vi "Get Peaks.vi"(8 "error in (no error)":errorcluster, 11 "Micron Hyperion Driver in":refnum<class "Micron Hyperion Driver.lvclass">) -> (0 "error out":errorcluster, 1 "Peaks per channel":i32[](array[numeric]), 2 "Peaks":dbl[](array[numeric]), 3 "Micron Hyperion Driver out":refnum<class "Micron Hyperion Driver.lvclass">)   [LabVIEW 2016, in "Micron Hyperion Driver.lvclass"]
uses:
  Micron Hyperion Driver.lvclass
  C:/github/NHMFL_Core/Libraries/Instruments/Micron Optics/Micron Optics Driver/Micron Optics Driver.lvclass
  C:/github/NHMFL_Core/Libraries/Instruments/Instrument Driver/Instrument Driver.lvclass
  Instrument Driver/Instrument Driver.lvclass/Instrument Driver.ctl
  Micron Optics Driver/Micron Optics Driver.lvclass/Micron Optics Driver.ctl
  Micron Optics Driver/Read Peaks buffer.vi
  Micron Optics Driver/Read Number of peaks.vi
  Instrument Driver/Read Cycle period.vi
  Micron Optics Driver/Read Micron Configuration.vi
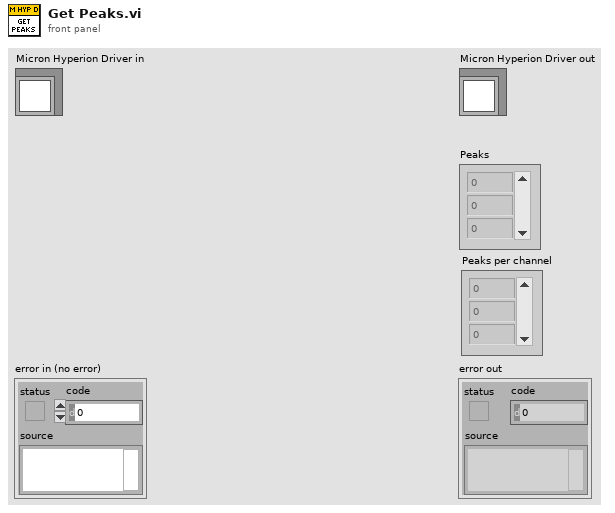
[diagram p1: front panel]
types:
  T1 = typedef "Micron optics configuration.ctl" = cluster{"Reference channel":i32, "Detection Setting IDs":u8[], "Address":string, "Stream and average":bool}
  T2 = typedef "h.Library.lvlib/h.ACQ.PeaksData.ctl" = cluster{"SN":u64, "Time Stamp (ns)":u64, "Header Version":u16, "Peaks Wvls, nm":T3[]}
  T3 = typedef "h.Library.lvlib/h.ACQ.PeaksWvl.ctl" = cluster{"Peak Wvls, nm":dbl[]}
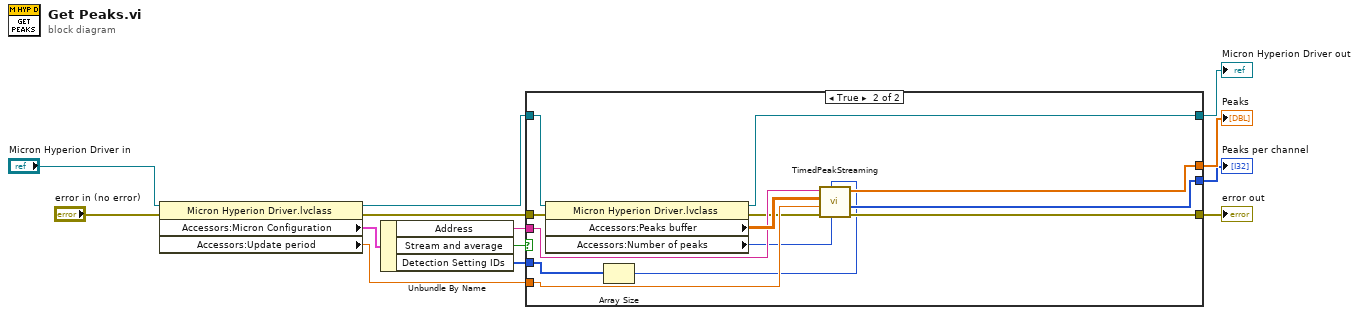
[diagram p0: block diagram]
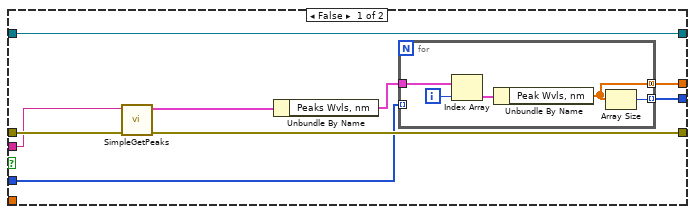
[diagram p2: hidden frame]
diagram:
  n1 = property class="Micron Hyperion Driver.lvclass"(reference="Micron Hyperion Driver in", error in="error in (no error)") -> (reference out=w5:refnum<class "Micron Hyperion Driver.lvclass">, error out=w13:errorcluster, "Accessors:Micron Configuration"=w12:T1, "Accessors:Update period"=w4:dbl)
  n2 = Unbundle By Name(w12) -> ("Address"=w7:string, "Stream and average"=w6:bool, "Detection Setting IDs"=w2:u8[])
  n3 = case shown="True" w6 {
    tunnel: w13 -> [w20 w34]
    tunnel: [w19 w32] -> w10
    tunnel: [w18 w36] -> w8
    tunnel: w7 -> [w17 w38]
    tunnel: w5 -> [w16 w40]
    tunnel: w4 -> [_ w37]
    tunnel: [w16 w33] -> w3
    tunnel: w2 -> [w15 w29]
    tunnel: [w14 w30] -> w1
    frame False {
      n4 = call "SimpleGetPeaks.vi"("Error In"=w20, "Address"=w17) -> ("Error Out"=w18:errorcluster, "Peaks Data"=w21:T2)  [unwired: 8 in]
      n5 = Unbundle By Name(w21) -> ("Peaks Wvls, nm"=w22:T3[])
      n6 = for {
        tunnel: w22 -> [w26]
        tunnel: [w24] -> w19 mode=concatenating
        tunnel: w15 -> [_] mode=indexing
        tunnel: [w23] -> w14 mode=indexing
        i -> [w25]
        n7 = Index Array(array=w26, index=w25) -> (element=w27:T3)
        n8 = Unbundle By Name(w27) -> ("Peak Wvls, nm"=w24:dbl[])
        n9 = Array Size(array=w24) -> (size(s)=w23:i32)
      }
    }
    frame True {
      n10 = property class="Micron Hyperion Driver.lvclass"(reference=w40, error in=w34) -> (reference out=w33:refnum<class "Micron Hyperion Driver.lvclass">, error out=w35:errorcluster, "Accessors:Peaks buffer"=w39:dbl[][], "Accessors:Number of peaks"=w31:i32)
      n11 = Array Size(array=w29) -> (size(s)=w28:i32)
      n12 = call "TimedPeakStreaming.vi"("Number of peaks"=w31, "Number of channels"=w28, "Error In"=w35, "Cycle period"=w37, "Peaks buffer"=w39, "Address"=w38) -> ("Error Out"=w36:errorcluster, "Peaks per channel"=w30:i32[], "Peaks"=w32:dbl[])  [unwired: 3 in]
    }
  }
  "error out" <- w8
  "Micron Hyperion Driver out" <- w3
  "Peaks" <- w10
  "Peaks per channel" <- w1
